vi "Calibration_sub.vi"(10 "Cluster in":T3={"String 2"="", "String"="", [], [], [], [], [], [], "mean"=0.0, "Test Type"=enum."Static Ramp", "Direction"=enum."CW", "Angle Target"=enum."45"}, 11 "mean":dbl) -> (3 "output cluster":T3)   [LabVIEW 2020]
uses:
  TESTtypedef UPDATED.ctl
  Angle Target NEW type def.ctl
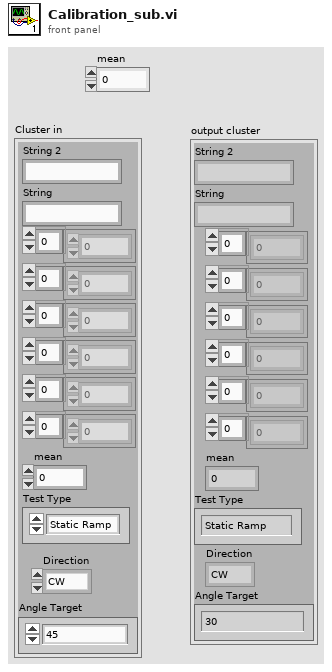
[diagram p1: front panel]
types:
  T1 = typedef "TESTtypedef UPDATED.ctl" = enum16{"Static Ramp", "Static Sine", "Dynamic"}
  T2 = typedef "Angle Target NEW type def.ctl" = enum16{"30", "45", "60", "75", "90"}
  T3 = cluster{"String 2":string, "String":string, dbl[], dbl[], dbl[], dbl[], dbl[], dbl[], "mean":dbl, "Test Type":T1, "Direction":enum16{"CW", "CCW"}, "Angle Target":T2}
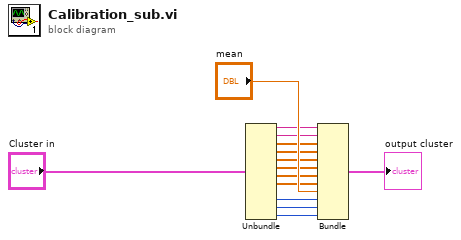
[diagram p0: block diagram]
diagram:
  n1 = Unbundle("Cluster in") -> ("String 2"=w6:string, "String"=w7:string, w8:dbl[], w9:dbl[], w10:dbl[], w11:dbl[], w5:dbl[], w12:dbl[], "Test Type"=w14:T1, "Direction"=w3:enum16{"CW", "CCW"}, "Angle Target"=w2:T2)  [unwired: 1 out]
  n2 = Bundle("String 2"=w6, "String"=w7, w8, w9, w10, w11, w5, w12, "mean"="mean", "Test Type"=w14, "Direction"=w3, "Angle Target"=w2) -> (→"output cluster":T3)  [unwired: 1 in]
